vi "Scheduler-uppaal.vi"(4 "Regional clusters, CL2":T1[](array[typedef])=[{"Regional set array"=[{"Lower lim"=20, "Upper lim"=27, "Equality req"=0, "First loop"=2, "Diff value"=-22, "Trigg plant"=1}, {"Lower lim"=7, "Upper lim"=21, "Equality req"=0, "First loop"=2, "Diff value"=-5, "Trigg plant"=2}, {"Lower lim"=0, "Upper lim"=27, "Equality req"=0, "First loop"=1, "Diff value"=-17, "Trigg plant"=2}, {"Lower lim"=20, "Upper lim"=27, "Equality req"=1, "First loop"=0, "Diff value"=0, "Trigg plant"=2}, {"Lower lim"=7, "Upper lim"=21, "Equality req"=0, "First loop"=2, "Diff value"=-2, "Trigg plant"=1}, {"Lower lim"=3, "Upper lim"=27, "Equality req"=0, "First loop"=1, "Diff value"=-17, "Trigg plant"=2}, {"Lower lim"=20, "Upper lim"=27, "Equality req"=0, "First loop"=1, "Diff value"=-20, "Trigg plant"=2}, {"Lower lim"=7, "Upper lim"=21, "Equality req"=0, "First loop"=0, "Diff value"=0, "Trigg plant"=1}, {"Lower lim"=7, "Upper lim"=27, "Equality req"=0, "First loop"=2, "Diff value"=-5, "Trigg plant"=2}, {"Lower lim"=27, "Upper lim"=27, "Equality req"=0, "First loop"=0, "Diff value"=0, "Trigg plant"=1}, {"Lower lim"=20, "Upper lim"=27, "Equality req"=0, "First loop"=2, "Diff value"=-26, "Trigg plant"=1}, {"Lower lim"=1, "Upper lim"=27, "Equality req"=0, "First loop"=2, "Diff value"=-5, "Trigg plant"=2}, {"Lower lim"=20, "Upper lim"=27, "Equality req"=0, "First loop"=1, "Diff value"=-2, "Trigg plant"=1}, {"Lower lim"=7, "Upper lim"=21, "Equality req"=0, "First loop"=1, "Diff value"=-2, "Trigg plant"=2}, {"Lower lim"=7, "Upper lim"=21, "Equality req"=0, "First loop"=2, "Diff value"=-2, "Trigg plant"=2}, {"Lower lim"=20, "Upper lim"=27, "Equality req"=0, "First loop"=2, "Diff value"=-25, "Trigg plant"=1}, {"Lower lim"=3, "Upper lim"=27, "Equality req"=0, "First loop"=2, "Diff value"=-5, "Trigg plant"=2}, {"Lower lim"=7, "Upper lim"=21, "Equality req"=0, "First loop"=0, "Diff value"=0, "Trigg plant"=2}, {"Lower lim"=3, "Upper lim"=27, "Equality req"=0, "First loop"=1, "Diff value"=-2, "Trigg plant"=2}, {"Lower lim"=5, "Upper lim"=27, "Equality req"=0, "First loop"=1, "Diff value"=-20, "Trigg plant"=2}, {"Lower lim"=7, "Upper lim"=27, "Equality req"=0, "First loop"=2, "Diff value"=-9, "Trigg plant"=2}, {"Lower lim"=25, "Upper lim"=25, "Equality req"=0, "First loop"=0, "Diff value"=0, "Trigg plant"=2}, {"Lower lim"=0, "Upper lim"=27, "Equality req"=0, "First loop"=2, "Diff value"=-2, "Trigg plant"=2}, {"Lower lim"=0, "Upper lim"=27, "Equality req"=0, "First loop"=1, "Diff value"=-2, "Trigg plant"=2}, {"Lower lim"=20, "Upper lim"=27, "Equality req"=0, "First loop"=1, "Diff value"=-2, "Trigg plant"=2}, {"Lower lim"=3, "Upper lim"=27, "Equality req"=0, "First loop"=2, "Diff value"=-2, "Trigg plant"=2}, {"Lower lim"=1, "Upper lim"=27, "Equality req"=0, "First loop"=1, "Diff value"=-2, "Trigg plant"=2}, {"Lower lim"=1, "Upper lim"=27, "Equality req"=0, "First loop"=2, "Diff value"=-2, "Trigg plant"=2}, {"Lower lim"=5, "Upper lim"=27, "Equality req"=0, "First loop"=1, "Diff value"=-17, "Trigg plant"=2}, {"Lower lim"=20, "Upper lim"=21, "Equality req"=0, "First loop"=1, "Diff value"=-17, "Trigg plant"=2}, {"Lower lim"=27, "Upper lim"=27, "Equality req"=0, "First loop"=0, "Diff value"=0, "Trigg plant"=2}, {"Lower lim"=20, "Upper lim"=27, "Equality req"=0, "First loop"=2, "Diff value"=-24, "Trigg plant"=1}, {"Lower lim"=27, "Upper lim"=27, "Equality req"=1, "First loop"=0, "Diff value"=0, "Trigg plant"=1}, {"Lower lim"=20, "Upper lim"=27, "Equality req"=0, "First loop"=2, "Diff value"=-2, "Trigg plant"=1}, {"Lower lim"=20, "Upper lim"=21, "Equality req"=0, "First loop"=1, "Diff value"=-20, "Trigg plant"=2}, {"Lower lim"=0, "Upper lim"=27, "Equality req"=0, "First loop"=2, "Diff value"=-5, "Trigg plant"=2}, {"Lower lim"=20, "Upper lim"=27, "Equality req"=0, "First loop"=2, "Diff value"=-23, "Trigg plant"=1}, {"Lower lim"=20, "Upper lim"=27, "Equality req"=1, "First loop"=0, "Diff value"=0, "Trigg plant"=1}, {"Lower lim"=1, "Upper lim"=27, "Equality req"=0, "First loop"=1, "Diff value"=-20, "Trigg plant"=2}, {"Lower lim"=17, "Upper lim"=17, "Equality req"=0, "First loop"=0, "Diff value"=0, "Trigg plant"=2}, {"Lower lim"=20, "Upper lim"=27, "Equality req"=0, "First loop"=2, "Diff value"=-28, "Trigg plant"=1}, {"Lower lim"=1, "Upper lim"=27, "Equality req"=0, "First loop"=1, "Diff value"=-17, "Trigg plant"=2}, {"Lower lim"=3, "Upper lim"=27, "Equality req"=0, "First loop"=1, "Diff value"=-20, "Trigg plant"=2}, {"Lower lim"=5, "Upper lim"=27, "Equality req"=0, "First loop"=1, "Diff value"=-2, "Trigg plant"=2}, {"Lower lim"=5, "Upper lim"=27, "Equality req"=0, "First loop"=2, "Diff value"=-2, "Trigg plant"=2}, {"Lower lim"=20, "Upper lim"=27, "Equality req"=0, "First loop"=2, "Diff value"=-27, "Trigg plant"=1}]}, ...(24 in all)], 5 "Regional clusters, CL1":T1[](array[typedef])=[{"Regional set array"=[{"Lower lim"=8, "Upper lim"=22, "Equality req"=1, "First loop"=0, "Diff value"=0, "Trigg plant"=2}, {"Lower lim"=25, "Upper lim"=32, "Equality req"=0, "First loop"=1, "Diff value"=-20, "Trigg plant"=2}, {"Lower lim"=4, "Upper lim"=26, "Equality req"=1, "First loop"=0, "Diff value"=0, "Trigg plant"=2}, {"Lower lim"=25, "Upper lim"=30, "Equality req"=0, "First loop"=2, "Diff value"=-2, "Trigg plant"=2}, {"Lower lim"=9, "Upper lim"=30, "Equality req"=1, "First loop"=0, "Diff value"=0, "Trigg plant"=2}, {"Lower lim"=25, "Upper lim"=32, "Equality req"=0, "First loop"=1, "Diff value"=-19, "Trigg plant"=2}, {"Lower lim"=3, "Upper lim"=27, "Equality req"=1, "First loop"=0, "Diff value"=0, "Trigg plant"=2}, {"Lower lim"=25, "Upper lim"=26, "Equality req"=0, "First loop"=2, "Diff value"=-5, "Trigg plant"=2}, {"Lower lim"=5, "Upper lim"=9, "Equality req"=1, "First loop"=0, "Diff value"=0, "Trigg plant"=2}, {"Lower lim"=8, "Upper lim"=25, "Equality req"=1, "First loop"=0, "Diff value"=0, "Trigg plant"=2}, {"Lower lim"=3, "Upper lim"=25, "Equality req"=1, "First loop"=0, "Diff value"=0, "Trigg plant"=2}, {"Lower lim"=4, "Upper lim"=26, "Equality req"=1, "First loop"=0, "Diff value"=0, "Trigg plant"=1}, {"Lower lim"=3, "Upper lim"=30, "Equality req"=1, "First loop"=0, "Diff value"=0, "Trigg plant"=2}, {"Lower lim"=3, "Upper lim"=7, "Equality req"=1, "First loop"=0, "Diff value"=0, "Trigg plant"=2}, {"Lower lim"=25, "Upper lim"=32, "Equality req"=0, "First loop"=1, "Diff value"=-8, "Trigg plant"=2}, {"Lower lim"=25, "Upper lim"=30, "Equality req"=0, "First loop"=2, "Diff value"=-22, "Trigg plant"=2}, {"Lower lim"=25, "Upper lim"=2, "Equality req"=0, "First loop"=0, "Diff value"=0, "Trigg plant"=2}, {"Lower lim"=5, "Upper lim"=28, "Equality req"=1, "First loop"=0, "Diff value"=0, "Trigg plant"=1}, {"Lower lim"=2, "Upper lim"=28, "Equality req"=1, "First loop"=0, "Diff value"=0, "Trigg plant"=2}, {"Lower lim"=25, "Upper lim"=32, "Equality req"=0, "First loop"=1, "Diff value"=-7, "Trigg plant"=2}, {"Lower lim"=8, "Upper lim"=12, "Equality req"=1, "First loop"=0, "Diff value"=0, "Trigg plant"=2}, {"Lower lim"=25, "Upper lim"=26, "Equality req"=0, "First loop"=2, "Diff value"=-12, "Trigg plant"=2}, {"Lower lim"=25, "Upper lim"=26, "Equality req"=0, "First loop"=2, "Diff value"=-22, "Trigg plant"=1}, {"Lower lim"=2, "Upper lim"=25, "Equality req"=1, "First loop"=0, "Diff value"=0, "Trigg plant"=2}, {"Lower lim"=2, "Upper lim"=26, "Equality req"=0, "First loop"=1, "Diff value"=-2, "Trigg plant"=2}, {"Lower lim"=17, "Upper lim"=17, "Equality req"=1, "First loop"=0, "Diff value"=0, "Trigg plant"=2}, {"Lower lim"=25, "Upper lim"=32, "Equality req"=0, "First loop"=1, "Diff value"=-26, "Trigg plant"=2}, {"Lower lim"=25, "Upper lim"=30, "Equality req"=0, "First loop"=2, "Diff value"=-25, "Trigg plant"=2}, {"Lower lim"=25, "Upper lim"=30, "Equality req"=0, "First loop"=2, "Diff value"=-4, "Trigg plant"=2}, {"Lower lim"=2, "Upper lim"=16, "Equality req"=1, "First loop"=0, "Diff value"=0, "Trigg plant"=2}, {"Lower lim"=25, "Upper lim"=32, "Equality req"=0, "First loop"=1, "Diff value"=-17, "Trigg plant"=2}, {"Lower lim"=2, "Upper lim"=26, "Equality req"=0, "First loop"=1, "Diff value"=-2, "Trigg plant"=1}, {"Lower lim"=7, "Upper lim"=22, "Equality req"=1, "First loop"=0, "Diff value"=0, "Trigg plant"=2}, {"Lower lim"=25, "Upper lim"=26, "Equality req"=0, "First loop"=2, "Diff value"=-2, "Trigg plant"=1}, {"Lower lim"=6, "Upper lim"=26, "Equality req"=1, "First loop"=0, "Diff value"=0, "Trigg plant"=2}, {"Lower lim"=7, "Upper lim"=20, "Equality req"=1, "First loop"=0, "Diff value"=0, "Trigg plant"=2}, {"Lower lim"=25, "Upper lim"=32, "Equality req"=0, "First loop"=1, "Diff value"=-14, "Trigg plant"=2}, {"Lower lim"=2, "Upper lim"=26, "Equality req"=0, "First loop"=2, "Diff value"=-12, "Trigg plant"=2}, {"Lower lim"=7, "Upper lim"=13, "Equality req"=1, "First loop"=0, "Diff value"=0, "Trigg plant"=2}, {"Lower lim"=6, "Upper lim"=20, "Equality req"=1, "First loop"=0, "Diff value"=0, "Trigg plant"=2}, {"Lower lim"=0, "Upper lim"=17, "Equality req"=1, "First loop"=0, "Diff value"=0, "Trigg plant"=2}, {"Lower lim"=25, "Upper lim"=32, "Equality req"=0, "First loop"=1, "Diff value"=-5, "Trigg plant"=2}, {"Lower lim"=5, "Upper lim"=22, "Equality req"=1, "First loop"=0, "Diff value"=0, "Trigg plant"=2}, {"Lower lim"=25, "Upper lim"=26, "Equality req"=0, "First loop"=2, "Diff value"=-22, "Trigg plant"=2}, {"Lower lim"=5, "Upper lim"=26, "Equality req"=1, "First loop"=0, "Diff value"=0, "Trigg plant"=1}, {"Lower lim"=5, "Upper lim"=29, "Equality req"=1, "First loop"=0, "Diff value"=0, "Trigg plant"=2}, {"Lower lim"=2, "Upper lim"=25, "Equality req"=1, "First loop"=0, "Diff value"=0, "Trigg plant"=1}, {"Lower lim"=25, "Upper lim"=30, "Equality req"=0, "First loop"=2, "Diff value"=-5, "Trigg plant"=2}, {"Lower lim"=4, "Upper lim"=18, "Equality req"=1, "First loop"=0, "Diff value"=0, "Trigg plant"=2}, {"Lower lim"=25, "Upper lim"=30, "Equality req"=0, "First loop"=2, "Diff value"=-25, "Trigg plant"=1}, {"Lower lim"=25, "Upper lim"=32, "Equality req"=0, "First loop"=1, "Diff value"=-24, "Trigg plant"=2}, {"Lower lim"=25, "Upper lim"=26, "Equality req"=0, "First loop"=2, "Diff value"=-25, "Trigg plant"=1}, {"Lower lim"=25, "Upper lim"=32, "Equality req"=0, "First loop"=1, "Diff value"=-2, "Trigg plant"=2}, {"Lower lim"=25, "Upper lim"=32, "Equality req"=0, "First loop"=1, "Diff value"=-23, "Trigg plant"=2}, {"Lower lim"=5, "Upper lim"=26, "Equality req"=1, "First loop"=0, "Diff value"=0, "Trigg plant"=2}, {"Lower lim"=2, "Upper lim"=26, "Equality req"=1, "First loop"=0, "Diff value"=0, "Trigg plant"=1}, {"Lower lim"=5, "Upper lim"=29, "Equality req"=1, "First loop"=0, "Diff value"=0, "Trigg plant"=1}, {"Lower lim"=3, "Upper lim"=17, "Equality req"=1, "First loop"=0, "Diff value"=0, "Trigg plant"=2}, {"Lower lim"=2, "Upper lim"=26, "Equality req"=0, "First loop"=2, "Diff value"=-2, "Trigg plant"=1}, {"Lower lim"=29, "Upper lim"=29, "Equality req"=1, "First loop"=0, "Diff value"=0, "Trigg plant"=2}, {"Lower lim"=25, "Upper lim"=26, "Equality req"=0, "First loop"=2, "Diff value"=-2, "Trigg plant"=2}, {"Lower lim"=5, "Upper lim"=12, "Equality req"=1, "First loop"=0, "Diff value"=0, "Trigg plant"=2}, {"Lower lim"=3, "Upper lim"=20, "Equality req"=1, "First loop"=0, "Diff value"=0, "Trigg plant"=2}, {"Lower lim"=25, "Upper lim"=30, "Equality req"=0, "First loop"=2, "Diff value"=-9, "Trigg plant"=2}, {"Lower lim"=25, "Upper lim"=32, "Equality req"=0, "First loop"=1, "Diff value"=-12, "Trigg plant"=2}, {"Lower lim"=5, "Upper lim"=32, "Equality req"=0, "First loop"=1, "Diff value"=-2, "Trigg plant"=1}, {"Lower lim"=2, "Upper lim"=26, "Equality req"=0, "First loop"=2, "Diff value"=-2, "Trigg plant"=2}, {"Lower lim"=3, "Upper lim"=29, "Equality req"=1, "First loop"=0, "Diff value"=0, "Trigg plant"=2}, {"Lower lim"=9, "Upper lim"=12, "Equality req"=1, "First loop"=0, "Diff value"=0, "Trigg plant"=2}, {"Lower lim"=25, "Upper lim"=32, "Equality req"=0, "First loop"=1, "Diff value"=-11, "Trigg plant"=2}, {"Lower lim"=2, "Upper lim"=26, "Equality req"=0, "First loop"=2, "Diff value"=-9, "Trigg plant"=2}, {"Lower lim"=9, "Upper lim"=14, "Equality req"=1, "First loop"=0, "Diff value"=0, "Trigg plant"=2}, {"Lower lim"=2, "Upper lim"=6, "Equality req"=1, "First loop"=0, "Diff value"=0, "Trigg plant"=2}, {"Lower lim"=4, "Upper lim"=8, "Equality req"=1, "First loop"=0, "Diff value"=0, "Trigg plant"=2}, {"Lower lim"=25, "Upper lim"=4, "Equality req"=0, "First loop"=0, "Diff value"=0, "Trigg plant"=2}, {"Lower lim"=1, "Upper lim"=15, "Equality req"=1, "First loop"=0, "Diff value"=0, "Trigg plant"=2}, {"Lower lim"=25, "Upper lim"=6, "Equality req"=0, "First loop"=0, "Diff value"=0, "Trigg plant"=2}, {"Lower lim"=2, "Upper lim"=24, "Equality req"=1, "First loop"=0, "Diff value"=0, "Trigg plant"=2}, {"Lower lim"=2, "Upper lim"=23, "Equality req"=1, "First loop"=0, "Diff value"=0, "Trigg plant"=1}, {"Lower lim"=25, "Upper lim"=30, "Equality req"=0, "First loop"=2, "Diff value"=-8, "Trigg plant"=2}, {"Lower lim"=2, "Upper lim"=26, "Equality req"=0, "First loop"=0, "Diff value"=0, "Trigg plant"=1}, {"Lower lim"=2, "Upper lim"=26, "Equality req"=1, "First loop"=0, "Diff value"=0, "Trigg plant"=2}, {"Lower lim"=1, "Upper lim"=25, "Equality req"=1, "First loop"=0, "Diff value"=0, "Trigg plant"=2}, {"Lower lim"=25, "Upper lim"=32, "Equality req"=0, "First loop"=1, "Diff value"=-21, "Trigg plant"=2}, {"Lower lim"=1, "Upper lim"=30, "Equality req"=0, "First loop"=0, "Diff value"=0, "Trigg plant"=2}, {"Lower lim"=5, "Upper lim"=30, "Equality req"=0, "First loop"=2, "Diff value"=-2, "Trigg plant"=1}, {"Lower lim"=1, "Upper lim"=27, "Equality req"=1, "First loop"=0, "Diff value"=0, "Trigg plant"=2}, {"Lower lim"=7, "Upper lim"=30, "Equality req"=1, "First loop"=0, "Diff value"=0, "Trigg plant"=2}, {"Lower lim"=5, "Upper lim"=27, "Equality req"=1, "First loop"=0, "Diff value"=0, "Trigg plant"=1}, {"Lower lim"=2, "Upper lim"=23, "Equality req"=1, "First loop"=0, "Diff value"=0, "Trigg plant"=2}, {"Lower lim"=2, "Upper lim"=24, "Equality req"=1, "First loop"=0, "Diff value"=0, "Trigg plant"=1}, {"Lower lim"=1, "Upper lim"=28, "Equality req"=1, "First loop"=0, "Diff value"=0, "Trigg plant"=2}, {"Lower lim"=25, "Upper lim"=26, "Equality req"=0, "First loop"=2, "Diff value"=-4, "Trigg plant"=2}, {"Lower lim"=25, "Upper lim"=3, "Equality req"=0, "First loop"=0, "Diff value"=0, "Trigg plant"=2}, {"Lower lim"=2, "Upper lim"=26, "Equality req"=0, "First loop"=0, "Diff value"=0, "Trigg plant"=2}, {"Lower lim"=2, "Upper lim"=32, "Equality req"=0, "First loop"=1, "Diff value"=-2, "Trigg plant"=1}, {"Lower lim"=0, "Upper lim"=27, "Equality req"=1, "First loop"=0, "Diff value"=0, "Trigg plant"=2}, {"Lower lim"=25, "Upper lim"=28, "Equality req"=0, "First loop"=0, "Diff value"=0, "Trigg plant"=2}, {"Lower lim"=25, "Upper lim"=32, "Equality req"=0, "First loop"=1, "Diff value"=-18, "Trigg plant"=2}, {"Lower lim"=7, "Upper lim"=21, "Equality req"=1, "First loop"=0, "Diff value"=0, "Trigg plant"=2}, {"Lower lim"=2, "Upper lim"=26, "Equality req"=0, "First loop"=2, "Diff value"=-8, "Trigg plant"=2}, {"Lower lim"=25, "Upper lim"=30, "Equality req"=0, "First loop"=2, "Diff value"=-12, "Trigg plant"=2}, {"Lower lim"=0, "Upper lim"=25, "Equality req"=1, "First loop"=0, "Diff value"=0, "Trigg plant"=2}, {"Lower lim"=1, "Upper lim"=23, "Equality req"=1, "First loop"=0, "Diff value"=0, "Trigg plant"=2}, {"Lower lim"=6, "Upper lim"=28, "Equality req"=1, "First loop"=0, "Diff value"=0, "Trigg plant"=2}, {"Lower lim"=12, "Upper lim"=12, "Equality req"=1, "First loop"=0, "Diff value"=0, "Trigg plant"=2}, {"Lower lim"=25, "Upper lim"=32, "Equality req"=0, "First loop"=1, "Diff value"=-9, "Trigg plant"=2}, {"Lower lim"=25, "Upper lim"=15, "Equality req"=0, "First loop"=0, "Diff value"=0, "Trigg plant"=2}, {"Lower lim"=6, "Upper lim"=30, "Equality req"=1, "First loop"=0, "Diff value"=0, "Trigg plant"=2}, {"Lower lim"=0, "Upper lim"=16, "Equality req"=1, "First loop"=0, "Diff value"=0, "Trigg plant"=2}, {"Lower lim"=7, "Upper lim"=11, "Equality req"=1, "First loop"=0, "Diff value"=0, "Trigg plant"=2}, {"Lower lim"=6, "Upper lim"=19, "Equality req"=1, "First loop"=0, "Diff value"=0, "Trigg plant"=2}, {"Lower lim"=5, "Upper lim"=16, "Equality req"=1, "First loop"=0, "Diff value"=0, "Trigg plant"=2}, {"Lower lim"=25, "Upper lim"=25, "Equality req"=1, "First loop"=0, "Diff value"=0, "Trigg plant"=1}, {"Lower lim"=25, "Upper lim"=32, "Equality req"=0, "First loop"=1, "Diff value"=-28, "Trigg plant"=2}, {"Lower lim"=6, "Upper lim"=30, "Equality req"=0, "First loop"=0, "Diff value"=0, "Trigg plant"=2}, {"Lower lim"=25, "Upper lim"=27, "Equality req"=0, "First loop"=0, "Diff value"=0, "Trigg plant"=2}, {"Lower lim"=6, "Upper lim"=10, "Equality req"=1, "First loop"=0, "Diff value"=0, "Trigg plant"=2}, {"Lower lim"=25, "Upper lim"=32, "Equality req"=0, "First loop"=1, "Diff value"=-6, "Trigg plant"=2}, {"Lower lim"=25, "Upper lim"=32, "Equality req"=0, "First loop"=1, "Diff value"=-27, "Trigg plant"=2}, {"Lower lim"=9, "Upper lim"=23, "Equality req"=1, "First loop"=0, "Diff value"=0, "Trigg plant"=2}, {"Lower lim"=6, "Upper lim"=13, "Equality req"=1, "First loop"=0, "Diff value"=0, "Trigg plant"=2}, {"Lower lim"=9, "Upper lim"=24, "Equality req"=1, "First loop"=0, "Diff value"=0, "Trigg plant"=2}, {"Lower lim"=25, "Upper lim"=26, "Equality req"=0, "First loop"=2, "Diff value"=-13, "Trigg plant"=2}, {"Lower lim"=4, "Upper lim"=21, "Equality req"=1, "First loop"=0, "Diff value"=0, "Trigg plant"=2}, {"Lower lim"=30, "Upper lim"=30, "Equality req"=0, "First loop"=0, "Diff value"=0, "Trigg plant"=1}, {"Lower lim"=5, "Upper lim"=27, "Equality req"=1, "First loop"=0, "Diff value"=0, "Trigg plant"=2}, {"Lower lim"=4, "Upper lim"=30, "Equality req"=1, "First loop"=0, "Diff value"=0, "Trigg plant"=2}, {"Lower lim"=30, "Upper lim"=30, "Equality req"=1, "First loop"=0, "Diff value"=0, "Trigg plant"=2}, {"Lower lim"=9, "Upper lim"=26, "Equality req"=1, "First loop"=0, "Diff value"=0, "Trigg plant"=2}, {"Lower lim"=8, "Upper lim"=23, "Equality req"=1, "First loop"=0, "Diff value"=0, "Trigg plant"=2}, {"Lower lim"=4, "Upper lim"=28, "Equality req"=1, "First loop"=0, "Diff value"=0, "Trigg plant"=2}, {"Lower lim"=5, "Upper lim"=25, "Equality req"=1, "First loop"=0, "Diff value"=0, "Trigg plant"=1}, {"Lower lim"=2, "Upper lim"=32, "Equality req"=0, "First loop"=1, "Diff value"=-2, "Trigg plant"=2}, {"Lower lim"=25, "Upper lim"=30, "Equality req"=0, "First loop"=2, "Diff value"=-13, "Trigg plant"=2}, {"Lower lim"=2, "Upper lim"=22, "Equality req"=1, "First loop"=0, "Diff value"=0, "Trigg plant"=1}, {"Lower lim"=8, "Upper lim"=21, "Equality req"=1, "First loop"=0, "Diff value"=0, "Trigg plant"=2}, {"Lower lim"=8, "Upper lim"=30, "Equality req"=1, "First loop"=0, "Diff value"=0, "Trigg plant"=2}, {"Lower lim"=30, "Upper lim"=30, "Equality req"=0, "First loop"=0, "Diff value"=0, "Trigg plant"=2}, {"Lower lim"=25, "Upper lim"=32, "Equality req"=0, "First loop"=1, "Diff value"=-16, "Trigg plant"=2}, {"Lower lim"=4, "Upper lim"=30, "Equality req"=0, "First loop"=0, "Diff value"=0, "Trigg plant"=2}, {"Lower lim"=3, "Upper lim"=26, "Equality req"=1, "First loop"=0, "Diff value"=0, "Trigg plant"=2}, {"Lower lim"=25, "Upper lim"=32, "Equality req"=0, "First loop"=1, "Diff value"=-15, "Trigg plant"=2}, {"Lower lim"=22, "Upper lim"=22, "Equality req"=1, "First loop"=0, "Diff value"=0, "Trigg plant"=1}, {"Lower lim"=9, "Upper lim"=13, "Equality req"=1, "First loop"=0, "Diff value"=0, "Trigg plant"=2}, {"Lower lim"=2, "Upper lim"=26, "Equality req"=0, "First loop"=2, "Diff value"=-5, "Trigg plant"=2}, {"Lower lim"=25, "Upper lim"=25, "Equality req"=0, "First loop"=0, "Diff value"=0, "Trigg plant"=1}, {"Lower lim"=8, "Upper lim"=15, "Equality req"=1, "First loop"=0, "Diff value"=0, "Trigg plant"=2}, {"Lower lim"=25, "Upper lim"=32, "Equality req"=0, "First loop"=1, "Diff value"=-4, "Trigg plant"=2}, {"Lower lim"=25, "Upper lim"=32, "Equality req"=0, "First loop"=1, "Diff value"=-25, "Trigg plant"=2}, {"Lower lim"=2, "Upper lim"=29, "Equality req"=1, "First loop"=0, "Diff value"=0, "Trigg plant"=2}, {"Lower lim"=5, "Upper lim"=30, "Equality req"=0, "First loop"=0, "Diff value"=0, "Trigg plant"=1}, {"Lower lim"=3, "Upper lim"=15, "Equality req"=1, "First loop"=0, "Diff value"=0, "Trigg plant"=2}, {"Lower lim"=8, "Upper lim"=13, "Equality req"=1, "First loop"=0, "Diff value"=0, "Trigg plant"=2}, {"Lower lim"=0, "Upper lim"=14, "Equality req"=1, "First loop"=0, "Diff value"=0, "Trigg plant"=2}, {"Lower lim"=25, "Upper lim"=32, "Equality req"=0, "First loop"=1, "Diff value"=-3, "Trigg plant"=2}, {"Lower lim"=25, "Upper lim"=10, "Equality req"=0, "First loop"=0, "Diff value"=0, "Trigg plant"=2}, {"Lower lim"=0, "Upper lim"=12, "Equality req"=1, "First loop"=0, "Diff value"=0, "Trigg plant"=2}, {"Lower lim"=2, "Upper lim"=22, "Equality req"=1, "First loop"=0, "Diff value"=0, "Trigg plant"=2}, {"Lower lim"=25, "Upper lim"=30, "Equality req"=0, "First loop"=2, "Diff value"=-7, "Trigg plant"=2}, {"Lower lim"=2, "Upper lim"=17, "Equality req"=1, "First loop"=0, "Diff value"=0, "Trigg plant"=2}, {"Lower lim"=7, "Upper lim"=29, "Equality req"=1, "First loop"=0, "Diff value"=0, "Trigg plant"=2}, {"Lower lim"=25, "Upper lim"=5, "Equality req"=0, "First loop"=0, "Diff value"=0, "Trigg plant"=2}, {"Lower lim"=25, "Upper lim"=32, "Equality req"=0, "First loop"=1, "Diff value"=-22, "Trigg plant"=2}, {"Lower lim"=3, "Upper lim"=26, "Equality req"=1, "First loop"=0, "Diff value"=0, "Trigg plant"=1}, {"Lower lim"=2, "Upper lim"=26, "Equality req"=0, "First loop"=2, "Diff value"=-4, "Trigg plant"=2}, {"Lower lim"=0, "Upper lim"=26, "Equality req"=1, "First loop"=0, "Diff value"=0, "Trigg plant"=2}, {"Lower lim"=2, "Upper lim"=19, "Equality req"=1, "First loop"=0, "Diff value"=0, "Trigg plant"=2}, {"Lower lim"=25, "Upper lim"=30, "Equality req"=0, "First loop"=2, "Diff value"=-2, "Trigg plant"=1}, {"Lower lim"=22, "Upper lim"=22, "Equality req"=0, "First loop"=0, "Diff value"=0, "Trigg plant"=1}, {"Lower lim"=25, "Upper lim"=7, "Equality req"=0, "First loop"=0, "Diff value"=0, "Trigg plant"=2}, {"Lower lim"=22, "Upper lim"=22, "Equality req"=1, "First loop"=0, "Diff value"=0, "Trigg plant"=2}, {"Lower lim"=25, "Upper lim"=32, "Equality req"=0, "First loop"=1, "Diff value"=-13, "Trigg plant"=2}, {"Lower lim"=7, "Upper lim"=24, "Equality req"=1, "First loop"=0, "Diff value"=0, "Trigg plant"=2}, {"Lower lim"=0, "Upper lim"=24, "Equality req"=1, "First loop"=0, "Diff value"=0, "Trigg plant"=2}, {"Lower lim"=1, "Upper lim"=18, "Equality req"=1, "First loop"=0, "Diff value"=0, "Trigg plant"=2}, {"Lower lim"=7, "Upper lim"=14, "Equality req"=1, "First loop"=0, "Diff value"=0, "Trigg plant"=2}, {"Lower lim"=0, "Upper lim"=22, "Equality req"=1, "First loop"=0, "Diff value"=0, "Trigg plant"=2}, {"Lower lim"=22, "Upper lim"=22, "Equality req"=0, "First loop"=0, "Diff value"=0, "Trigg plant"=2}, {"Lower lim"=5, "Upper lim"=30, "Equality req"=1, "First loop"=0, "Diff value"=0, "Trigg plant"=1}, {"Lower lim"=7, "Upper lim"=12, "Equality req"=1, "First loop"=0, "Diff value"=0, "Trigg plant"=2}, {"Lower lim"=6, "Upper lim"=21, "Equality req"=1, "First loop"=0, "Diff value"=0, "Trigg plant"=2}, {"Lower lim"=25, "Upper lim"=32, "Equality req"=0, "First loop"=1, "Diff value"=-10, "Trigg plant"=2}, {"Lower lim"=9, "Upper lim"=16, "Equality req"=1, "First loop"=0, "Diff value"=0, "Trigg plant"=2}, {"Lower lim"=5, "Upper lim"=19, "Equality req"=1, "First loop"=0, "Diff value"=0, "Trigg plant"=2}, {"Lower lim"=25, "Upper lim"=26, "Equality req"=0, "First loop"=2, "Diff value"=-9, "Trigg plant"=2}, {"Lower lim"=25, "Upper lim"=30, "Equality req"=0, "First loop"=2, "Diff value"=-22, "Trigg plant"=1}, {"Lower lim"=6, "Upper lim"=23, "Equality req"=1, "First loop"=0, "Diff value"=0, "Trigg plant"=2}, {"Lower lim"=9, "Upper lim"=25, "Equality req"=1, "First loop"=0, "Diff value"=0, "Trigg plant"=2}, {"Lower lim"=9, "Upper lim"=30, "Equality req"=0, "First loop"=0, "Diff value"=0, "Trigg plant"=2}, {"Lower lim"=5, "Upper lim"=30, "Equality req"=0, "First loop"=2, "Diff value"=-22, "Trigg plant"=1}, {"Lower lim"=4, "Upper lim"=20, "Equality req"=1, "First loop"=0, "Diff value"=0, "Trigg plant"=2}, {"Lower lim"=5, "Upper lim"=30, "Equality req"=1, "First loop"=0, "Diff value"=0, "Trigg plant"=2}]}, ...(4 in all)], 6 "Index array, CL2":i32[](array[numeric])=[0, 0, 0, 0, 0, 0, 0, 6, 8, 10, 2, 12, 7, 1, 13, 14, 17, 9, 21, 6, 23, 11, 0, 20, 18, 4, 5, 15, 22, 19, 16], 7 "Index array, CL1":i32[](array[numeric])=[0, 0, 0, 0, 0, 0, 0, 0, 0, 0, 0, 0, 0, 0, 0, 0, 0, 0, 0, 0, 0, 0, 0, 0, 0, 0, 0, 0, 3, 2, 1], 8 "Clock, plant 2":i32=-2, 9 "Region, plant 2":i32=7, 10 "Clock, plant 1":i32, 11 "Region, plant 1":i32=27) -> (0 "Clock 2":i32=-2, 1 "Clock 1":i32, 2 "Trigger?":bool=TRUE, 3 "Plant to trigg":enum16{"Plant 1", "Plant 2"}(ring)=enum."Plant 2")   [LabVIEW 2016]
uses:
  Strategy_regional_cluster.ctl
  Strategy_regional_set.ctl
  <vilib>/Platform/TimedLoop/XDataNode/timing_clust.ctl
  <vilib>/Platform/TimedLoop/XDataNode/nitl_modes.ctl
  <vilib>/Platform/TimedLoop/XDataNode/wakeup.ctl
  <vilib>/Platform/TimedLoop/XDataNode/XDataNode.xnode
  <vilib>/Platform/TimedLoop/XDataNode/XDNodeRunTimeDep.lvlib
panel:
  # "The regions are provided by the plants/main loop;\nthe scheduler follows the UPPAAL-generated\nstrategy to decide the next steps to be taken"
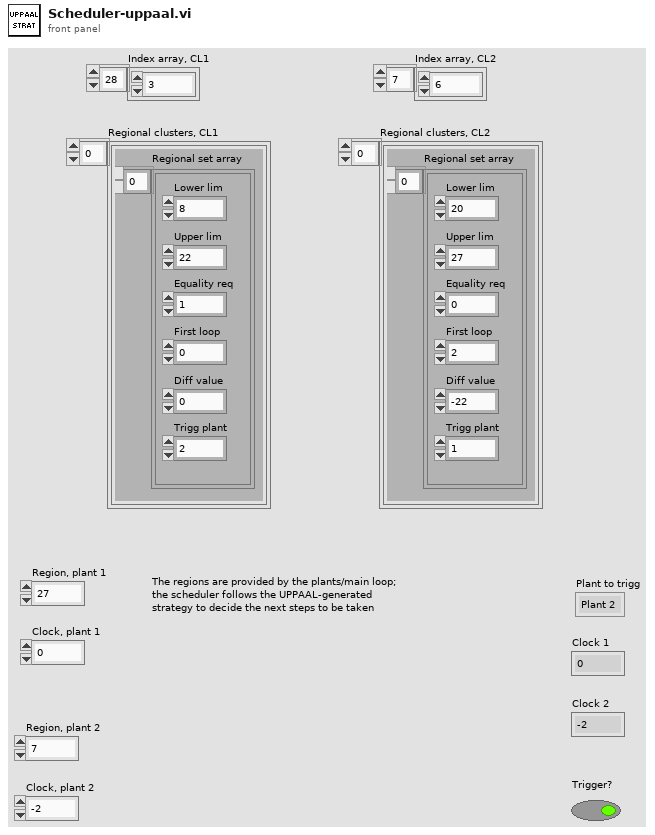
[diagram p1: front panel]
types:
  T1 = typedef "Strategy_regional_cluster.ctl" = cluster{"Regional set array":T2[]}
  T2 = typedef "Strategy_regional_set.ctl" = cluster{"Lower lim":i32, "Upper lim":i32, "Equality req":i32, "First loop":i32, "Diff value":i32, "Trigg plant":i32}
  T3 = typedef "XDNodeRunTimeDep.lvlib/timing_clust.ctl" = cluster{"Expected End [f-1]":u64, "Actual End [f-1]":u64, "Finished Late? [f-1]":bool, "Expected End [i-1]":u64, "Actual End [i-1]":u64, "Finished Late? [i-1]":bool, "Expected Start [i]":u64, "Actual Start [i]":u64, "Expected Start [f]":u64, "Actual Start [f]":u64, "Source Name":string, "Structure Name":string, "Period":i64, "Deadline":i64, "Offset":i64, "Start":i64, "Priority":i32, "Timeout":i32, "Mode":T4, "Wakeup Reason":T5, "Error":errorcluster, "Source Type":string, "Secondary Source Type":string, "Global End Time":u64, "Global Start Time":u64, "Frame Duration":u64, "Iteration Duration":u64, "Assigned CPU":i32, "I/O Scan Engine Mode":u32}
  T4 = typedef "XDNodeRunTimeDep.lvlib/nitl_modes.ctl" = enum32{"No Change", "Process missed periods, maintain original phase", "Discard missed periods, maintain original phase", "Process missed periods, ignore original phase", "Discard missed periods, ignore original phase"}
  T5 = typedef "XDNodeRunTimeDep.lvlib/wakeup.ctl" = enum32{"Normal", "Aborted", "Asynchronous wakeup", "Timing source error", "Timed loop error", "Timeout"}
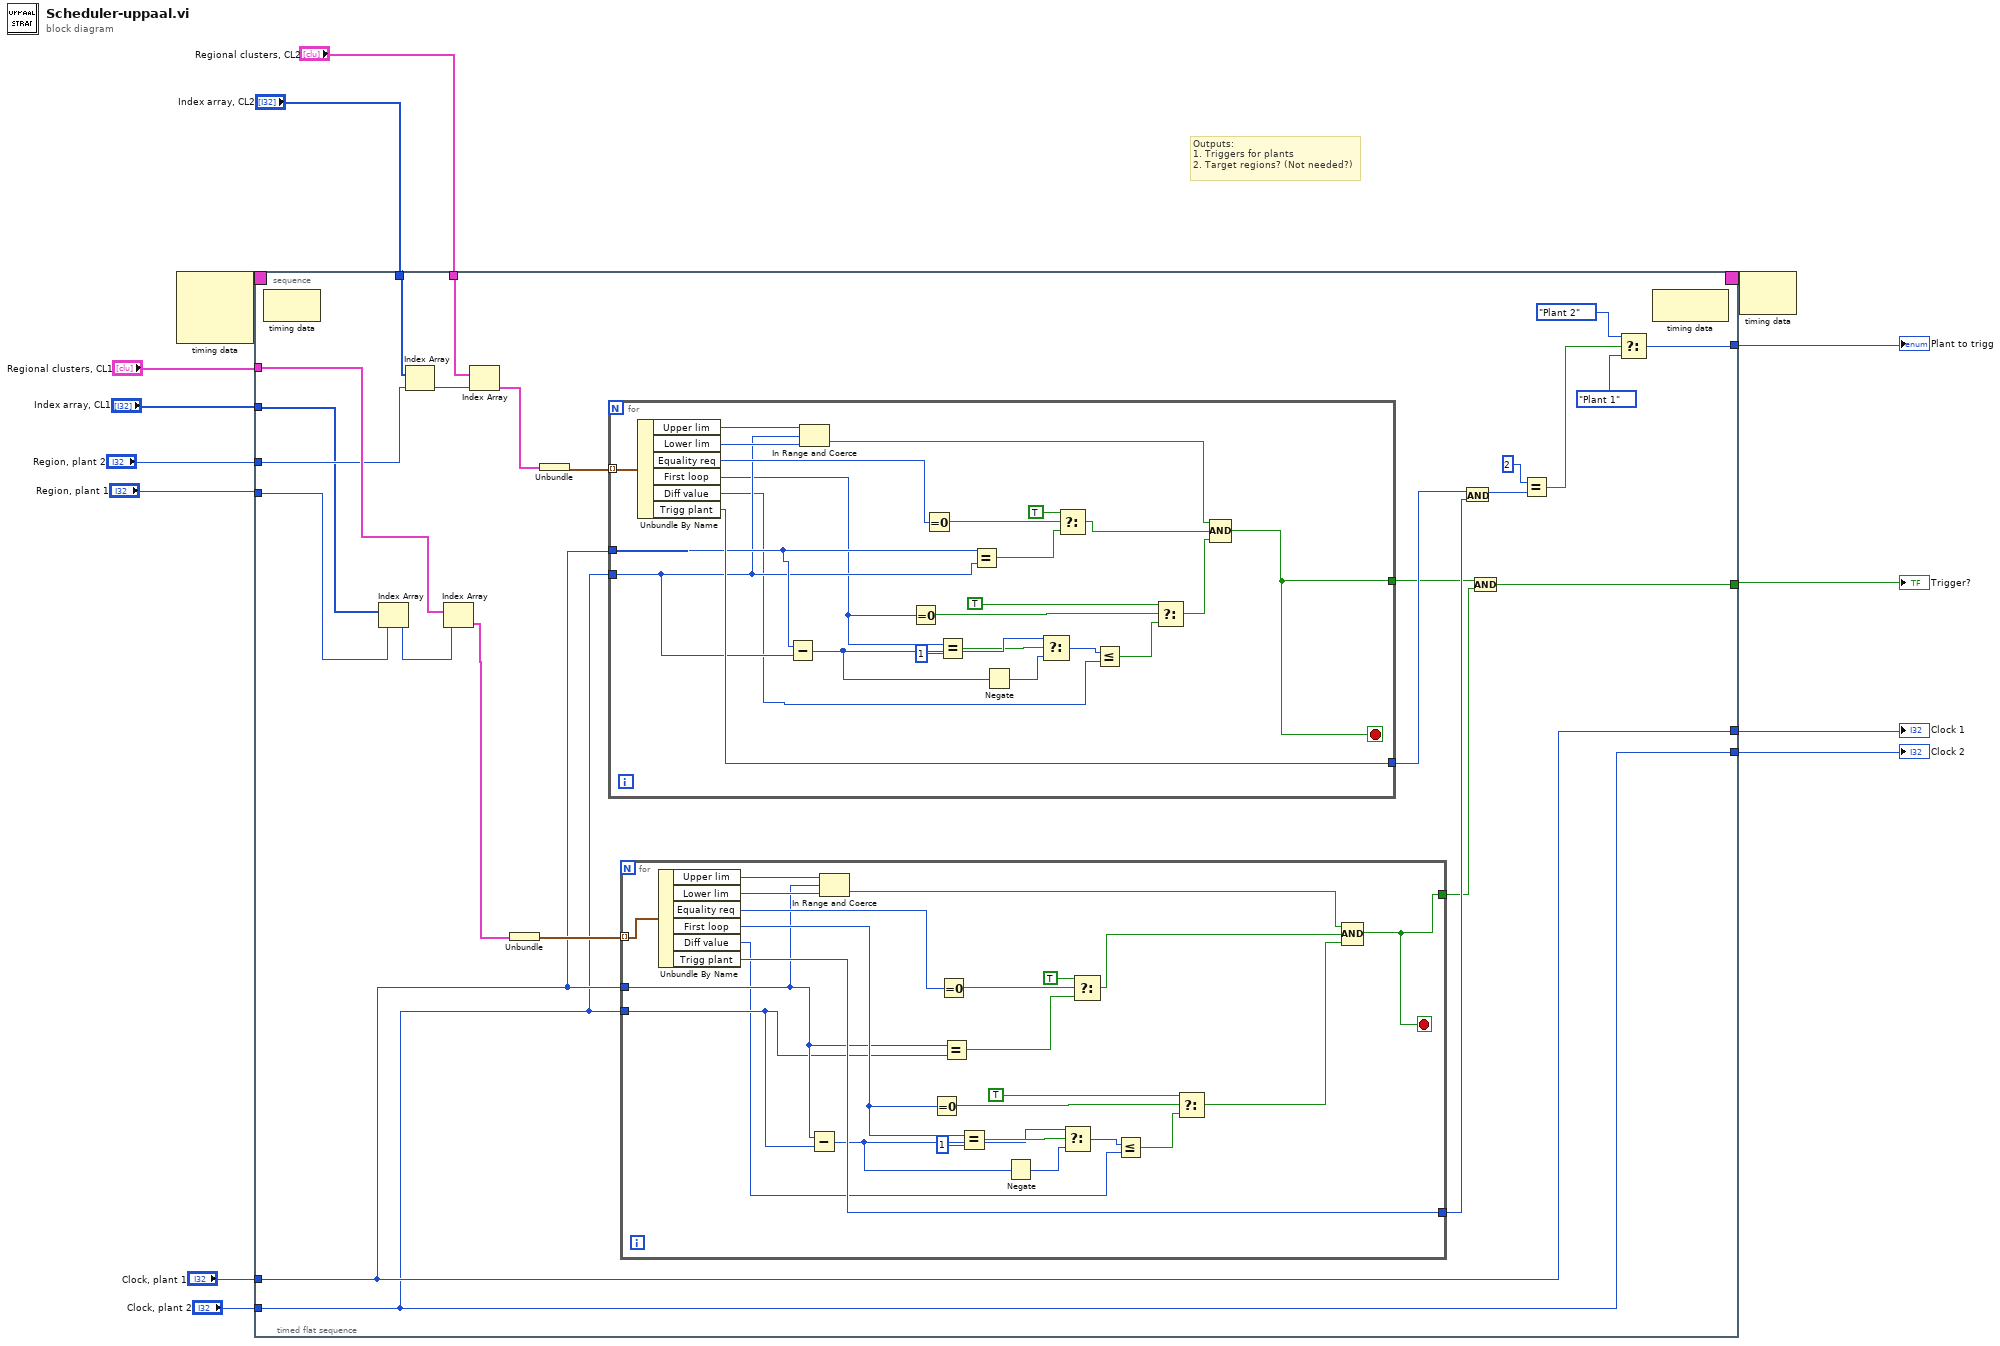
[diagram p0: block diagram]
diagram:
  # "Outputs:\n1. Triggers for plants\n2. Target regions? (Not needed?)"
  n1 = node-c288() -> (w14:T3)  [unwired: 3 in]
  n2 = timed-sequence {
    timing: w14 -> [_]
    timing-out: [_] -> w13
    tunnel: "Clock, plant 1" -> [w17]
    tunnel: "Clock, plant 2" -> [w18]
    tunnel: [w26] -> w10
    tunnel: [w25] -> w9
    tunnel: "Region, plant 2" -> [w24]
    tunnel: "Region, plant 1" -> [w23]
    tunnel: "Index array, CL1" -> [w21]
    tunnel: "Index array, CL2" -> [w22]
    tunnel: "Regional clusters, CL1" -> [w20]
    tunnel: "Regional clusters, CL2" -> [w19]
    tunnel: [w16] -> w2
    tunnel: [w15] -> w1
    n3 = timed-flat-sequence {
      tunnel: [w32] -> w26
      tunnel: [w51] -> w25
      tunnel: w24 -> [w43]
      tunnel: w23 -> [w48]
      tunnel: w22 -> [w44]
      tunnel: w21 -> [w37]
      tunnel: w20 -> [w47]
      tunnel: w19 -> [w42]
      tunnel: w18 -> [w29]
      tunnel: w17 -> [w30]
      tunnel: [w30] -> w16
      tunnel: [w29] -> w15
      n4 = node-c288() -> ()  [unwired: 1 in, 1 out]
      n5 = Index Array(array=w37, index=w48) -> (element=w46:i32)
      n6 = Index Array(array=w44, index=w43) -> (element=w45:i32)
      n7 = Index Array(array=w47, index=w46) -> (element=w41:T1)
      n8 = Index Array(array=w42, index=w45) -> (element=w40:T1)
      n9 = Unbundle(w41) -> ("Regional set array"=w38:T2[])
      n10 = Unbundle(w40) -> ("Regional set array"=w39:T2[])
      n11 = for {
        tunnel: w39 -> [w99] mode=indexing
        tunnel: w30 -> [w83]
        tunnel: w29 -> [w82]
        tunnel: [w96] -> w36
        tunnel: [w76] -> w28
        stop <- w76 stop-if-true
        n12 = Unbundle By Name(w99) -> ("Upper lim"=w98:i32, "Lower lim"=w97:i32, "Equality req"=w93:i32, "First loop"=w81:i32, "Diff value"=w80:i32, "Trigg plant"=w96:i32)
        n13 = Subtract(x=w83, y=w82) -> (x-y=w88:i32)
        n14 = In Range and Coerce(upper limit=w98, x=w82, lower limit=w97) -> (In Range?=w79:bool)  [unwired: 1 out]
        n15 = Equal To 0?(x=w81) -> (x = 0?=w84:bool)
        n16 = Equal To 0?(x=w93) -> (x = 0?=w94:bool)
        n17 = Equal?(x=w81, y=1) -> (x = y?=w87:bool)
        n18 = Equal?(x=w83, y=w82) -> (x = y?=w92:bool)
        n19 = Negate(x=w88) -> (-x=w89:i32)
        n20 = Select(t=w88, s=w87, f=w89) -> (s? t:f=w90:i32)
        n21 = Select(t=TRUE, s=w94, f=w92) -> (s? t:f=w78:bool)
        n22 = Less Or Equal?(x=w90, y=w80) -> (x <= y?=w91:bool)
        n23 = Select(t=TRUE, s=w84, f=w91) -> (s? t:f=w77:bool)
        n24 = Compound Arithmetic op=AND(w79, w78, w77) -> (w76:bool)
      }
      n25 = for {
        tunnel: w38 -> [w73] mode=indexing
        tunnel: w29 -> [w61]
        tunnel: w30 -> [w62]
        tunnel: [w72] -> w35
        tunnel: [w52] -> w27
        stop <- w52 stop-if-true
        n26 = Unbundle By Name(w73) -> ("Upper lim"=w74:i32, "Lower lim"=w75:i32, "Equality req"=w71:i32, "First loop"=w66:i32, "Diff value"=w57:i32, "Trigg plant"=w72:i32)
        n27 = Subtract(x=w62, y=w61) -> (x-y=w60:i32)
        n28 = In Range and Coerce(upper limit=w74, x=w62, lower limit=w75) -> (In Range?=w53:bool)  [unwired: 1 out]
        n29 = Equal To 0?(x=w66) -> (x = 0?=w67:bool)
        n30 = Equal To 0?(x=w71) -> (x = 0?=w70:bool)
        n31 = Equal?(x=w62, y=w61) -> (x = y?=w69:bool)
        n32 = Equal?(x=w66, y=1) -> (x = y?=w63:bool)
        n33 = Negate(x=w60) -> (-x=w59:i32)
        n34 = Select(t=w60, s=w63, f=w59) -> (s? t:f=w58:i32)
        n35 = Select(t=TRUE, s=w70, f=w69) -> (s? t:f=w54:bool)
        n36 = Less Or Equal?(x=w58, y=w57) -> (x <= y?=w56:bool)
        n37 = Select(t=TRUE, s=w67, f=w56) -> (s? t:f=w55:bool)
        n38 = Compound Arithmetic op=AND(w53, w54, w55) -> (w52:bool)
      }
      n39 = And(x=w36, y=w35) -> (x .and. y?=w34:i32)
      n40 = And(x=w28, y=w27) -> (x .and. y?=w32:bool)
      n41 = Equal?(x=2, y=w34) -> (x = y?=w31:bool)
      n42 = Select(t=enum16{"Plant 1", "Plant 2"}."Plant 2" ("Plants"), s=w31, f=enum16{"Plant 1", "Plant 2"}."Plant 1" ("Plants")) -> (s? t:f=w51:enum16{"Plant 1", "Plant 2"})
      n43 = node-c288() -> ()  [unwired: 1 in, 1 out]
    }
  }
  "Clock 1" <- w2
  "Clock 2" <- w1
  "Trigger?" <- w10
  "Plant to trigg" <- w9
  n44 = node-c288(w13) -> ()  [unwired: 1 out]
